vi "Custom_Generate_pseudo_unique_filename.vi"(7 "VI":refnum<vi>, 9 "Suffix":string, 10 "Optional iterator":i32, 11 "file type(.jpg)":T1) -> (1 "root filename":string, 2 "temp directory":path, 3 "generated path":path)   [LabVIEW 2019]
uses:
  <vilib>/printing/ReportDocExtensions.llb/File_types_for_reports.ctl
  <vilib>/Utility/NIReport.llb/NI_ReportGenerationCore.lvlib
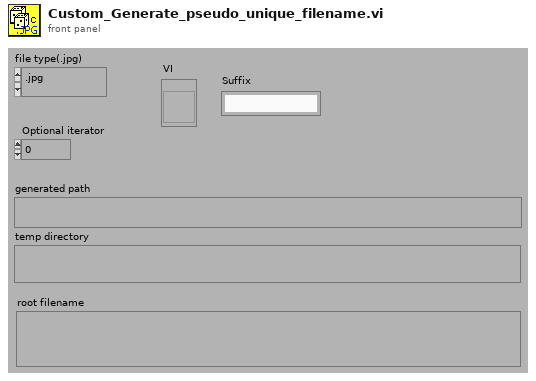
[diagram p1: front panel]
types:
  T1 = typedef "NI_ReportGenerationCore.lvlib/File_types_for_reports.ctl" = enum16{".jpg", ".png", ".html", ".gif"}
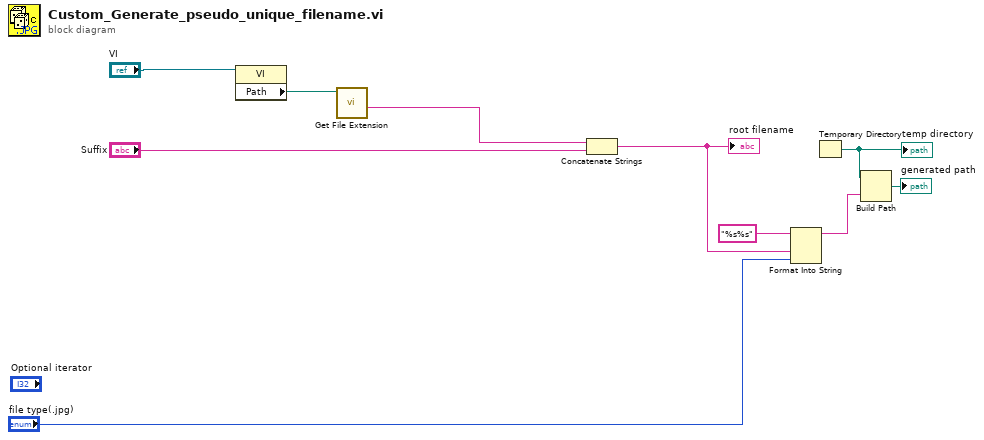
[diagram p0: block diagram]
diagram:
  n1 = property class="VI"(reference="VI") -> ("Path"=w4:path)  [unwired: 1 in, 2 out]
  n2 = call <vilib>:"Get File Extension.vi"("file"=w4) -> ("filename without extension"=w3:string)  [unwired: 6 in, 4 out]
  n3 = Concatenate Strings(w3, "Suffix") -> (w2:string)
  "root filename" <- w2
  n4 = Format Into String(format string="%s%s", w2, "file type(.jpg)") -> (resulting string=w6:string)  [unwired: 2 in, 1 out]
  n5 = Temporary Directory() -> (w10:path)
  "temp directory" <- w10
  n6 = Build Path(base path=w10, name or relative path=w6) -> (appended path=→"generated path":path)
